vi "confirmation_input.vi"(7 "caller":refnum<vi>, 8 "error in (no error)":errorcluster, 11 "configuration":T2) -> (0 "error out":errorcluster, 3 "dialog_selection":T1=enum."button_2")   [LabVIEW 2015, in "lv-dialog-interfaces.lvlib"]
uses:
  lv-dialog-interfaces.lvlib
  <userlib>/antonio-alexander/lv-dialog/api/v1/public/_controls/selection.ctl
  private/_controls/dialog_type.ctl
  private/_controls/hmi_references.ctl
  private/_controls/configuration.ctl
  <vilib>/event_ctls.llb/eventvkey.ctl
  <userlib>/antonio-alexander/lv-dialog/api/v1/v1.lvlib
panel:
  out "confirmation_dialog":string
  in  "confirmation_input":string
  in  "button 1":bool
  in  "button_2":bool
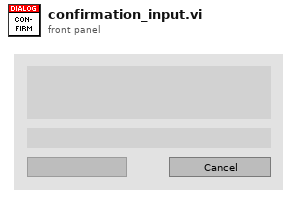
[diagram p1: front panel]
types:
  T1 = typedef "lv-dialog.lvlib/v1.lvlib/selection.ctl" = enum16{"null", "panel_closed", "button_1", "button_2", "button_3", "cancelled"}
  T2 = cluster{"dialog_text":string, "confirmation_text":string, "boolean_text_1":string, "boolean_text_2":string}
  T3 = typedef "lv-dialog-interfaces.lvlib/dialog_type.ctl" = enum16{"null", "one_button", "two_button", "three_button", "confirmation", "busy_wait", "error", "busy_wait_embed", "combo_box", "data_entry_string", "data_entry_numeric"}
  T4 = typedef "lv-dialog-interfaces.lvlib/configuration.ctl" = cluster{"dialog_text":string, "boolean_text_1":string, "boolean_text_2":string, "boolean_text_3":string, "inner_color":u32, "outer_color":u32, "wait_s":dbl, "error_status":bool, "error_source":string, "error_details":string, "string []":string[], "custom_entry":bool, "confirmation_text":string}
  T5 = typedef "lv-dialog-interfaces.lvlib/hmi_references.ctl" = cluster{"vi_reference":refnum<vi>, "caller":refnum<vi>, "dialog":refnum<vi>, "button_1":refnum<vi>, "button_2":refnum<vi>, "button_3":refnum<vi>, "busy":refnum<vi>, "error_glyph":refnum<vi>, "error_source":refnum<vi>, "error_text":refnum<vi>, "combo_box":refnum<vi>}
  T6 = typedef "eventvkey.ctl" = enum16{"ASCII", "Enter", "Return", "Shift", "Ctrl", "Alt", "Cmd", "Opt", "Caps", "NumLock", "Clear", "Break", "Up", "Down", "Left", "Right", "Insert", "Delete", "Home", "End", "PageUp", "PageDown", "Escape", "Help", "Pause", "ScrollLock", "F1", "F2", "F3", "F4", "F5", "F6", "F7", "F8", "F9", "F10", "F11", "F12", "F13", "F14", "F15", "F16", "F17", "F18", "F19", "F20", "F21", "F22", "F23", "F24", "Play", "VolumeUp", "VolumeDown", "Mute", "Two Byte Char"}
  T7 = enum8{"Enabled", "Disabled", "Disabled and Grayed Out"}
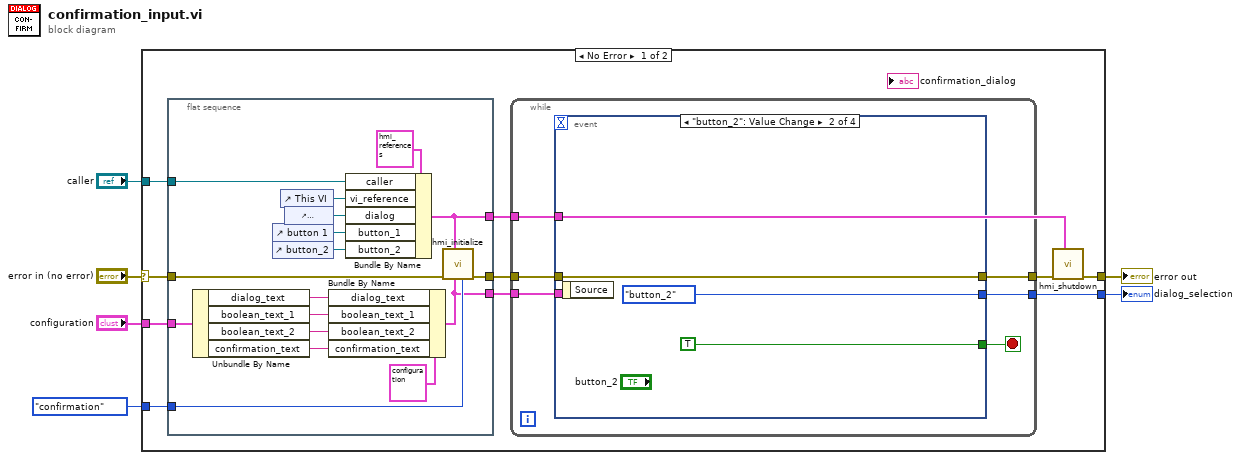
[diagram p0: block diagram]
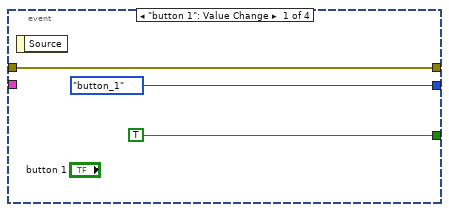
[diagram p2: hidden frame]
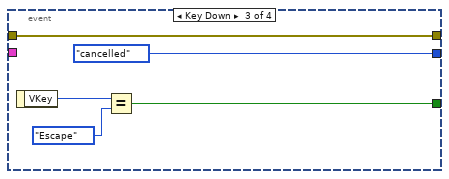
[diagram p3: hidden frame]
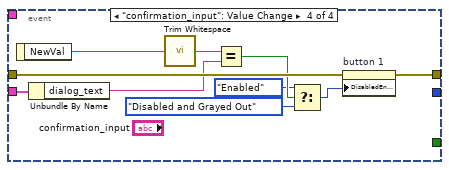
[diagram p4: hidden frame]
diagram:
  n1 = case shown="No Error" "error in (no error)" {
    selector: "error in (no error)" -> [w14 w61]
    tunnel: [w15 w61] -> w6
    tunnel: [w13 _] -> w1
    tunnel: "caller" -> [w12 _]
    tunnel: "configuration" -> [w11 _]
    tunnel: dialog_type."confirmation" ("dialog_type") -> [w10 _]
    frame No Error {
      n2 = flat-sequence {
        tunnel: w14 -> [w26]
        tunnel: w11 -> [w22]
        tunnel: [w27] -> w9
        tunnel: [w21] -> w8
        tunnel: w12 -> [w31]
        tunnel: w10 -> [w25]
        tunnel: [w24] -> w7
        frame #0 {
          n3 = Unbundle By Name(w22) -> ("dialog_text"=w20:string, "boolean_text_1"=w19:string, "boolean_text_2"=w18:string, "confirmation_text"=w17:string)
          n4 = control-ref of="button 1"() -> (w30:refnum<vi>)
          n5 = control-ref of="button_2"() -> (w29:refnum<vi>)
          n6 = control-ref of="This VI"() -> (w32:refnum<vi>)
          n7 = control-ref of="confirmation_dialog"() -> (w28:refnum<vi>)
          n8 = Bundle By Name(cluster=T4 {"dialog_text"="", "boolean_text_1"="", "boolean_text_2"="", "boolean_text_3"="", "inner_color"=16711680, "outer_color"=6618880, "wait_s"=nan, "error_status"=FALSE, "error_source"="", "error_details"="", "string []"=[], "custom_entry"=FALSE, "confirmation_text"=""} ("configuration"), "dialog_text"=w20, "boolean_text_1"=w19, "boolean_text_2"=w18, "confirmation_text"=w17) -> (w21:T4)
          n9 = Bundle By Name(cluster=T5 {"vi_reference"=refnum, "caller"=refnum, "dialog"=refnum, "button_1"=refnum, "button_2"=refnum, "button_3"=refnum, "busy"=refnum, "error_glyph"=refnum, "error_source"=refnum, "error_text"=refnum, "combo_box"=refnum} ("references"), "caller"=w31, "vi_reference"=w32, "dialog"=w28, "button_1"=w30, "button_2"=w29) -> (w24:T5)
          n10 = call "hmi_initialize.vi"("dialog_type"=w25, "configuration"=w21, "references"=w24, "error in (no error)"=w26) -> ("error out"=w27:errorcluster)  [unwired: 7 in]
        }
      }
      n11 = while {
        tunnel: w9 -> [w36]
        tunnel: [w39] -> w13
        tunnel: w8 -> [w37]
        tunnel: [w35] -> w16
        tunnel: w7 -> [w34]
        stop <- w38 stop-if-true
        n12 = event shown="[1] \"button_2\": Value Change" {
          selector: _ -> [_ _ _ _]
          dyn-events: _ -> [_ _ _ _]
          timeout: _ -> [_ _ _ _]
          tunnel: [selection."button_1" ("dialog_selection") selection."button_2" ("dialog_selection") selection."cancelled" ("dialog_selection") _] -> w39
          tunnel: [TRUE TRUE w48 _] -> w38
          tunnel: w37 -> [_ _ _ w51]
          tunnel: w36 -> [w41 w43 w49 w59]
          tunnel: [w41 w43 w49 w57] -> w35
          tunnel: w34 -> [_ _ _ _]
          event "button 1": Value Change {
            n13 = event-data() -> ()  [unwired: 1 in, 1 out]
          }
          event "button_2": Value Change {
            n14 = event-data() -> ()  [unwired: 1 in, 1 out]
          }
          event Key Down {
            n15 = event-data() -> ("VKey"=w47:T6)  [unwired: 1 in]
            n16 = Equal?(x=w47, y=eventvkey."Escape" ("VKey")) -> (x = y?=w48:bool)
          }
          event "confirmation_input": Value Change {
            n17 = event-data() -> ("NewVal"=w58:string)  [unwired: 1 in]
            n18 = Unbundle By Name(w51) -> ("dialog_text"=w52:string)
            n19 = call <vilib>:"Trim Whitespace.vi"("string"=w58) -> ("trimmed string"=w60:string)  [unwired: 1 in]
            n20 = Equal?(x=w60, y=w52) -> (x = y?=w55:bool)
            n21 = Select(t=T7."Enabled" ("Disabled"), s=w55, f=T7."Disabled and Grayed Out" ("Disabled")) -> (s? t:f=w56:T7)
            n22 = property on="button 1" class="Bool"(error in=w59, "DisabledEnum"=w56) -> (error out=w57:errorcluster)  [unwired: 1 in, 1 out]
          }
        }
      }
      n23 = call "hmi_shutdown.vi"("references"=w7, "error in (no error)"=w16) -> ("error out"=w15:errorcluster)  [unwired: 9 in]
    }
    frame Error {
    }
  }
  "error out" <- w6
  "dialog_selection" <- w1
